vi "coutout.vi"(0 "总数输入":dbl, 1 "OK输入":dbl, 2 "OK":bool, 5 "error in (no error)":errorcluster caption="错误输入（无错误）") -> (14 "总数输出":dbl, 15 "OK输出":dbl, 16 "NG输出":dbl, 17 "良率":dbl, 19 "error out":errorcluster caption="错误输出")   [LabVIEW 2018]
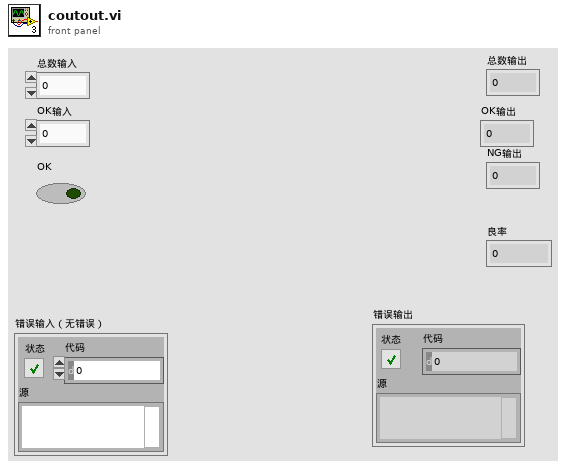
[diagram p1: front panel]
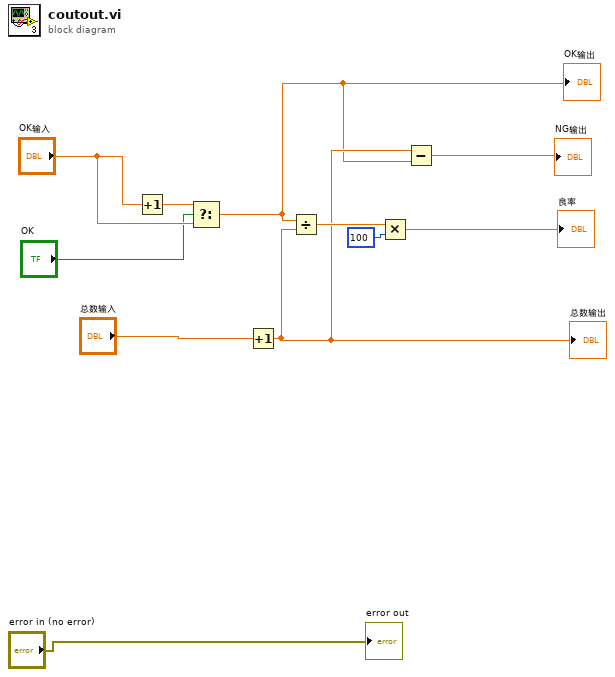
[diagram p0: block diagram]
diagram:
  n1 = Increment(x="OK输入") -> (x+1=w4:dbl)
  n2 = Select(t=w4, s="OK", f="OK输入") -> (s? t:f=w1:dbl)
  "OK输出" <- w1
  n3 = Increment(x="总数输入") -> (x+1=w2:dbl)
  "总数输出" <- w2
  n4 = Divide(x=w1, y=w2) -> (x/y=w8:dbl)
  n5 = Multiply(x=w8, y=100) -> (x*y=→"良率":dbl)
  n6 = Subtract(x=w2, y=w1) -> (x-y=→"NG输出":dbl)
  "error out" <- "error in (no error)"
